vi "BeamGage Chart.vi"() -> ()   [LabVIEW 2019]
uses:
  C:/Program Files/Spiricon/BeamGage Professional/Spiricon.Automation.dll
  Spiricon.Automation.dll
  C:/Program Files/Spiricon/BeamGage Professional/Spiricon.BeamGage.Automation.dll
  Spiricon.BeamGage.Automation.dll
panel:
  out "Status":i32(ring)=4 items=["NOT_SUPPORTED", "FAILED", "CALIBRATING", "READY", "BEAM_DETECTED"]
  out "2D Intensity Graph":dbl[][](graph)
  out "1D Profile - Peak Location Y - Waveform Graph":dbl[](graph)
  out "Height":dbl
  out "Width":dbl
  out "Peak Loc Y":dbl
  out "Peak Loc X":dbl
  in  "START_STOP":bool
  in  "ULTRACAL":bool
  out "Total and Peak Power - Waveform Chart":cluster{"Total":dbl, "Peak":dbl}(graph)
  in  "STOP SERVER":bool
  # "Block laser beam and \nclick Ultracal to calibrate"
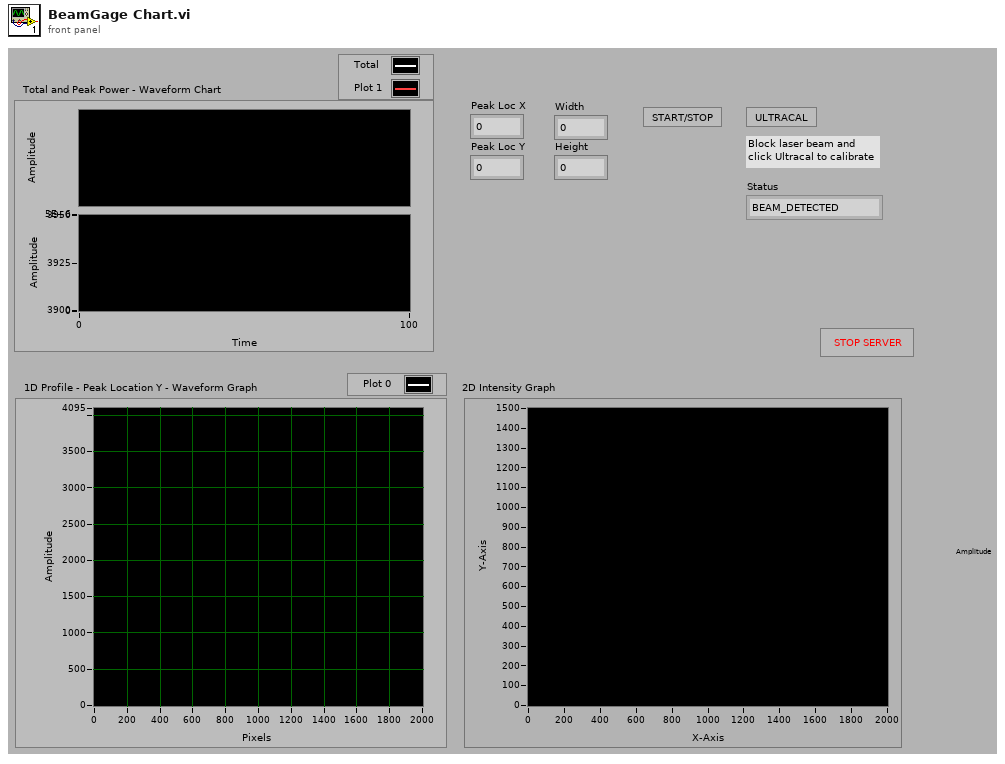
[diagram p1: front panel]
types:
  T1 = cluster{"Total":dbl, "Peak":dbl, "Peak X":dbl, "Peak Y":dbl, "Width":dbl, "Height":dbl, "DoubleData":dbl[], "Scale Multiplier":dbl}
  T2 = cluster{"notifier out":refnum<notifier>, "new reference":refnum<k24>}
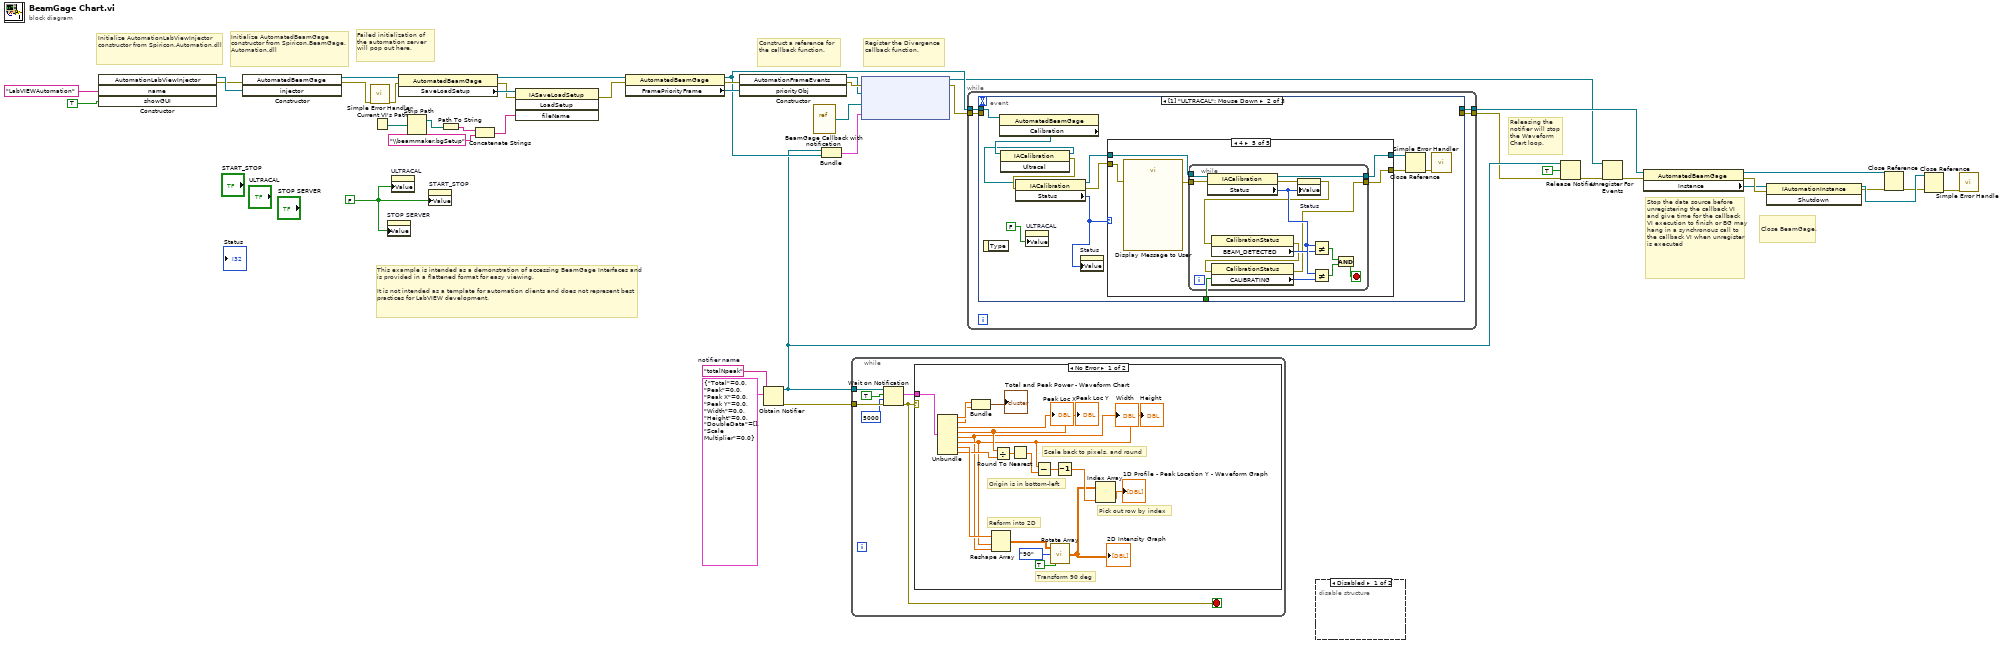
[diagram p0: block diagram]
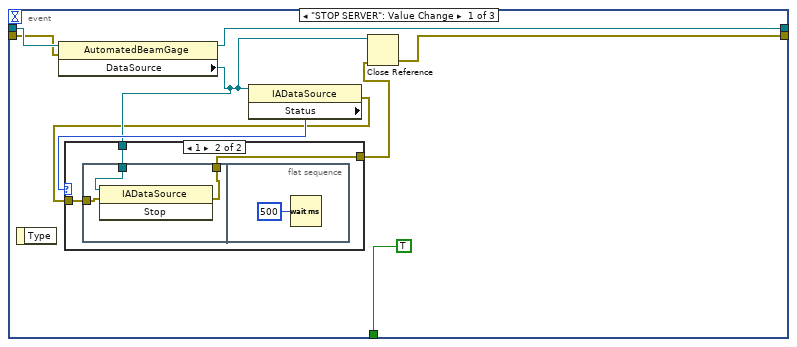
[diagram p3: hidden frame]
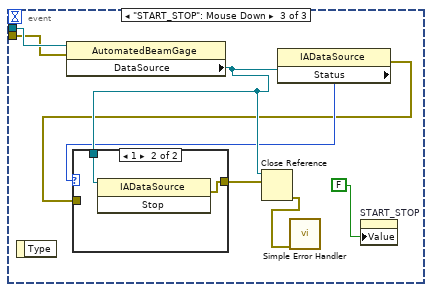
[diagram p9: hidden frame]
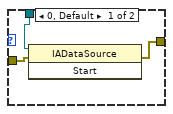
[diagram p10: hidden frame]
diagram:
  w39 = FALSE ("stop")
  w42 = "totalNpeak"  # notifier name
  # "Initialize AutomationLabViewInjector constructor from Spiricon.Automation.dll"
  # "Failed initialization of the automation server will pop out here."
  # "This example is intended as a demonstration of accessing BeamGage Interfaces and is provided in a flattened format for easy viewing.\n\nIt is not intended as a template for automation clients and does not represent best practices for LabVIEW development."
  # "Stop the data source before unregistering the callback VI  and give time for the callback VI execution to finish or BG may hang in a synchronous call to the callback VI when unregister is executed"
  # "Releasing the notifier will stop the Waveform Chart loop."
  # "Close BeamGage."
  # "Initialize AutomatedBeamGage constructor from Spiricon.BeamGage.Automation.dll"
  # "Register the Divergence callback function."
  # "Construct a reference for the callback function."
  n1 = constructor class="AutomationLabViewInjector"("name"="LabVIEWAutomation" ("Name"), "showGUI"=TRUE ("LaunchUI")) -> (reference out=w4:refnum<k24>, error out=w1:errorcluster)  [unwired: 3 in, 3 out]
  n2 = constructor class="AutomatedBeamGage"(error in=w1, "injector"=w4) -> (reference out=w35:refnum<k24>, error out=w6:errorcluster)  [unwired: 2 in, 2 out]
  n3 = call <vilib>:"Simple Error Handler.vi"("error in (no error)"=w6) -> ("error out"=w5:errorcluster)  [unwired: 4 in, 4 out]
  n4 = Current VI's Path() -> (path=w28:path)
  n5 = property on="STOP SERVER" class="Bool (strict)"("Value"=w39) -> ()  [unwired: 2 in, 2 out]
  n6 = property on="ULTRACAL" class="Bool (strict)"("Value"=w39) -> ()  [unwired: 2 in, 2 out]
  n7 = property class="AutomatedBeamGage"(reference=w35, error in=w5) -> (reference out=w31:refnum<k24>, error out=w33:errorcluster, "SaveLoadSetup"=w34:refnum<k24>)
  n8 = Strip Path(path=w28) -> (stripped path=w27:path)  [unwired: 1 out]
  n9 = property on="START_STOP" class="Bool (strict)"("Value"=w39) -> ()  [unwired: 2 in, 2 out]
  n10 = Path To String(path=w27) -> (string=w30:string)
  n11 = Concatenate Strings(w30, "\\beammaker.bgSetup" ("string")) -> (w26:string)
  n12 = invoke class="IASaveLoadSetup" method="LoadSetup"(reference=w34, error in=w33, "fileName"=w26) -> (error out=w32:errorcluster)  [unwired: 1 in, 3 out]
  n13 = property class="AutomatedBeamGage"(reference=w31, error in=w32) -> (reference out=w36:refnum<k24>, error out=w37:errorcluster, "FramePriorityFrame"=w38:refnum<k24>)
  n14 = constructor class="AutomationFrameEvents"(error in=w37, "priorityObj"=w38) -> (reference out=w24:refnum<k24>, error out=w25:errorcluster)  [unwired: 2 in, 2 out]
  n15 = Obtain Notifier(name (unnamed)=w42, notification data type=T1 {"Total"=0.0, "Peak"=0.0, "Peak X"=0.0, "Peak Y"=0.0, "Width"=0.0, "Height"=0.0, "DoubleData"=[], "Scale Multiplier"=0.0}) -> (notifier out=w9:refnum<notifier>, error out=w40:errorcluster)  [unwired: 2 in, 1 out]
  n16 = vi-ref "BeamGage Callback with notification.vi"() -> ("vi reference"=w21:refnum<vi>)
  n17 = Bundle("notifier out"=w9, "new reference"=w36) -> (w22:T2)  [unwired: 1 in]
  n18 = while {
    tunnel: w9 -> [w48]
    tunnel: w40 -> [w46]
    stop <- w44 stop-if-true
    n19 = Wait on Notification(notifier=w48, ignore previous (F)=TRUE, timeout in ms (-1)=5000, error in (no error)=w46) -> (notification=w47:T1, error out=w44:errorcluster)  [unwired: 2 out]
    n20 = case shown="No Error" w44 {
      tunnel: w47 -> [w67 _]
      frame No Error {
        # "Transform 90 deg"
        # "Scale back to pixels, and round"
        # "Pick out row by index"
        # "Reform into 2D"
        # "Origin is in bottom-left"
        n21 = Unbundle(w67) -> ("Total"=w66:dbl, "Peak"=w65:dbl, "Peak X"=→"Peak Loc X":dbl, "Peak Y"=w59:dbl, "Width"=w53:dbl, "Height"=w54:dbl, "DoubleData"=w61:dbl[], "Scale Multiplier"=w55:dbl)
        "Peak Loc Y" <- w59
        "Width" <- w53
        "Height" <- w54
        n22 = Bundle("Total"=w66, "Peak"=w65) -> (→"Total and Peak Power - Waveform Chart":cluster{"Total":dbl, "Peak":dbl})  [unwired: 1 in]
        n23 = Reshape Array(w61, w54, w53) -> (w52:dbl[][])
        n24 = Divide(x=w59, y=w55) -> (x/y=w60:dbl)
        n25 = Round To Nearest(number=w60) -> (nearest integer value=w57:dbl)
        n26 = Subtract(x=w54, y=w57) -> (x-y=w58:dbl)
        n27 = call "Rotate Array.vi"("Rotation Orientation"=TRUE, "Rotation"=enum8{"90", "180", "270"}."90", "Array"=w52) -> ("Rotated 2D Array"=w51:dbl[][])
        "2D Intensity Graph" <- w51
        n28 = Decrement(x=w58) -> (x-1=w56:dbl)
        n29 = Index Array(array=w51, index (col)=w56) -> (element=→"1D Profile - Peak Location Y - Waveform Graph":dbl[])  [unwired: 1 in]
      }
      frame Error {
        # "Don't update chart when an error occurs."
      }
    }
  }
  n30 = node(w25, w24, w21, w22) -> (w10:refnum<k27>, w23:errorcluster)  [unwired: 1 in]
  n31 = while {
    tunnel: [w72] -> w11
    tunnel: w36 -> [w71]
    tunnel: w23 -> [w69]
    tunnel: [w68] -> w8
    stop <- w70 stop-if-true
    n32 = event shown="[1] \"ULTRACAL\": Mouse Down" {
      selector: _ -> [_ _ _]
      dyn-events: _ -> [_ _ _]
      timeout: _ -> [_ _ _]
      tunnel: w71 -> [w79 w99 w131]
      tunnel: [w78 _ _] -> w72
      tunnel: [TRUE ("stop") _ _] -> w70
      tunnel: w69 -> [w77 _ w130]
      tunnel: [w80 _ _] -> w68
      event "STOP SERVER": Value Change {
        n33 = event-data() -> ()  [unwired: 1 in, 1 out]
        n34 = property class="AutomatedBeamGage"(reference=w79, error in=w77) -> (reference out=w78:refnum<k24>, "DataSource"=w75:refnum<k24>)  [unwired: 1 out]
        n35 = property class="IADataSource"(reference=w75) -> (error out=w73:errorcluster, "Status"=w76:i32)  [unwired: 1 in, 1 out]
        n36 = case shown="1" w76 {
          tunnel: w75 -> [_ w85]
          tunnel: [w82 w84] -> w74
          tunnel: w73 -> [w82 w83]
          frame 0, Default {
          }
          frame 1 {
            n37 = flat-sequence {
              tunnel: w85 -> [w88]
              tunnel: [w87] -> w84
              tunnel: w83 -> [w86]
              frame #0 {
                n38 = invoke class="IADataSource" method="Stop"(reference=w88, error in=w86) -> (error out=w87:errorcluster)  [unwired: 1 in, 2 out]
              }
              frame #1 {
                n39 = Wait (ms)(milliseconds to wait=u32 500) -> ()  [unwired: 1 out]
              }
            }
          }
        }
        n40 = Close Reference(reference=w75, error in (no error)=w74) -> (error out=w80:errorcluster)
      }
      event "ULTRACAL": Mouse Down {
        n41 = event-data() -> ()  [unwired: 1 in, 1 out]
        n42 = property class="AutomatedBeamGage"(reference=w99) -> ("Calibration"=w98:refnum<k24>)  [unwired: 1 in, 2 out]
        n43 = invoke class="IACalibration" method="Ultracal"(reference=w98) -> (reference out=w96:refnum<k24>, error out=w97:errorcluster)  [unwired: 2 in, 1 out]
        n44 = property class="IACalibration"(reference=w96, error in=w97) -> (reference out=w95:refnum<k24>, error out=w94:errorcluster, "Status"=w93:i32)
        n45 = property on="ULTRACAL" class="Bool (strict)"("Value"=FALSE ("stop")) -> ()  [unwired: 2 in, 2 out]
        n46 = property on="Status" class="Ring (strict)"("Value"=w93) -> ()  [unwired: 2 in, 2 out]
        n47 = case shown="4" w93 {
          tunnel: [w101 w103 w105 w107 w109] -> w90
          tunnel: [w102 w104 w106 w108 w111] -> w91
          tunnel: w95 -> [w102 w104 w106 w108 w112]
          tunnel: w94 -> [w101 w103 w105 w107 w113]
          frame 0, Default {
          }
          frame 1 {
          }
          frame 2 {
          }
          frame 3 {
          }
          frame 4 {
            n48 = call "Display Message to User"("error in (no error)"=w113) -> ("error out"=w110:errorcluster)  [unwired: 9 in, 1 out]
            n49 = while {
              tunnel: w112 -> [w126]
              tunnel: [w125] -> w111
              tunnel: w110 -> [w124]
              tunnel: [w114] -> w109
              stop <- w122 stop-if-true
              n50 = property class="IACalibration"(reference=w126, error in=w124) -> (reference out=w125:refnum<k24>, error out=w123:errorcluster, "Status"=w119:i32)
              n51 = property on="Status" class="Ring (strict)"(error in=w123, "Value"=w119) -> (error out=w118:errorcluster)  [unwired: 1 in, 1 out]
              n52 = property class="CalibrationStatus"(error in=w118) -> (error out=w115:errorcluster, "BEAM_DETECTED"=w117:i32)  [unwired: 1 in, 1 out]
              n53 = property class="CalibrationStatus"(error in=w115) -> (error out=w114:errorcluster, "CALIBRATING"=w116:i32)  [unwired: 1 in, 1 out]
              n54 = Not Equal?(x=w119, y=w117) -> (x != y?=w120:bool)
              n55 = Not Equal?(x=w119, y=w116) -> (x != y?=w121:bool)
              n56 = And(x=w120, y=w121) -> (x .and. y?=w122:bool)
            }
          }
        }
        n57 = Close Reference(reference=w91, error in (no error)=w90) -> (error out=w92:errorcluster)
        n58 = call <vilib>:"Simple Error Handler.vi"("error in (no error)"=w92) -> ()  [unwired: 4 in, 5 out]
      }
      event "START_STOP": Mouse Down {
        n59 = event-data() -> ()  [unwired: 1 in, 1 out]
        n60 = property class="AutomatedBeamGage"(reference=w131, error in=w130) -> ("DataSource"=w129:refnum<k24>)  [unwired: 2 out]
        n61 = property class="IADataSource"(reference=w129) -> (error out=w127:errorcluster, "Status"=w128:i32)  [unwired: 1 in, 1 out]
        n62 = case shown="1" w128 {
          tunnel: [w135 w139] -> w133
          tunnel: w129 -> [w137 w138]
          tunnel: w127 -> [w136 _]
          frame 0, Default {
            n63 = invoke class="IADataSource" method="Start"(reference=w137, error in=w136) -> (error out=w135:errorcluster)  [unwired: 1 in, 2 out]
          }
          frame 1 {
            n64 = invoke class="IADataSource" method="Stop"(reference=w138) -> (error out=w139:errorcluster)  [unwired: 2 in, 2 out]
          }
        }
        n65 = Close Reference(reference=w129, error in (no error)=w133) -> (error out=w132:errorcluster)
        n66 = call <vilib>:"Simple Error Handler.vi"("error in (no error)"=w132) -> ()  [unwired: 4 in, 5 out]
        n67 = property on="START_STOP" class="Bool (strict)"("Value"=FALSE ("stop")) -> ()  [unwired: 2 in, 2 out]
      }
    }
  }
  n68 = disable-structure shown="Disabled" {
    frame Disabled {
    }
    frame Enabled {
    }
  }
  n69 = Release Notifier(notifier=w9, force destroy? (F)=TRUE, error in (no error)=w8) -> (error out=w12:errorcluster)  [unwired: 2 out]
  n70 = Unregister For Events(event registration refnum=w10, error in=w12) -> (error out=w16:errorcluster)
  n71 = property class="AutomatedBeamGage"(reference=w11, error in=w16) -> (reference out=w15:refnum<k24>, error out=w17:errorcluster, "Instance"=w14:refnum<k24>)
  n72 = invoke class="IAutomationInstance" method="Shutdown"(reference=w14, error in=w17) -> (reference out=w19:refnum<k24>, error out=w13:errorcluster)  [unwired: 1 in, 1 out]
  n73 = Close Reference(reference=w15, error in (no error)=w13) -> (error out=w18:errorcluster)
  n74 = Close Reference(reference=w19, error in (no error)=w18) -> (error out=w7:errorcluster)
  n75 = call <vilib>:"Simple Error Handler.vi"("error in (no error)"=w7) -> ()  [unwired: 4 in, 5 out]
